vi "geschwindigkeit.vi"() -> ()   [LabVIEW 2013]
panel:
  out "x'":dbl
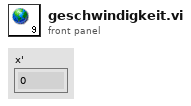
[diagram p1: front panel]
diagram:
